vi "Formic Queen.vi"(8 "error in (no error)":errorcluster, 9 "SelfID":i32, 10 "Map":i32[](array[numeric]), 11 "Mother in":refnum<class "Formics.lvclass">) -> (0 "error out":errorcluster, 1 "Direction":T1, 2 "Action":T2, 3 "Mother out":refnum<class "Formics.lvclass">, 4 "Replicated Class":refnum<class "Formics.lvclass">)   [LabVIEW 2015, in "Formics.lvclass"]
uses:
  Formics.lvclass
  Type Defs/Action Enum.ctl
  Type Defs/Direction Enum.ctl
  Formics.lvclass/Formics.ctl
  SquareStatus.ctl
  Formic Types.ctl
  Type Defs/SB Type Defs.lvlib
  Common/Common.lvlib
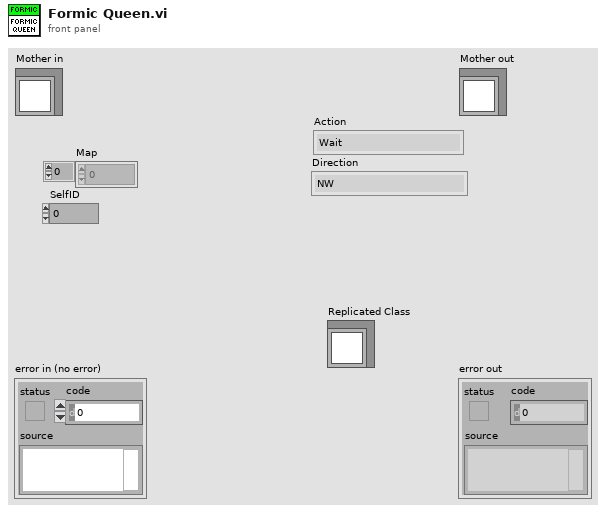
[diagram p1: front panel]
types:
  T1 = typedef "SB Type Defs.lvlib/Direction Enum.ctl" = enum16{"NW", "N", "NE", "E", "SE", "S", "SW", "W"}
  T2 = typedef "SB Type Defs.lvlib/Action Enum.ctl" = enum16{"Wait", "Move", "Attack", "Replicate"}
  T3 = typedef "Formics.lvclass/Formic Types.ctl" = enum16{"Queen Bee", "Protector Bee", "Daughter Bee", "Worker Bee", "Coward"}
  T4 = typedef "Formics.lvclass/SquareStatus.ctl" = cluster{"ID":i32, "Heartbeat":bool, "MyPosition":cluster{"X":i32, "Y":i32}}
  T5 = typedef "Formics.lvclass/Kamikaze DVR.ctl" = refnum<data-value>
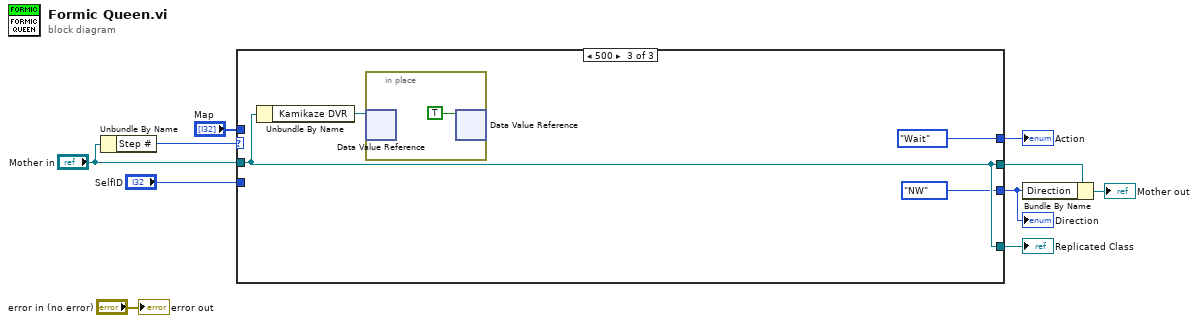
[diagram p0: block diagram]
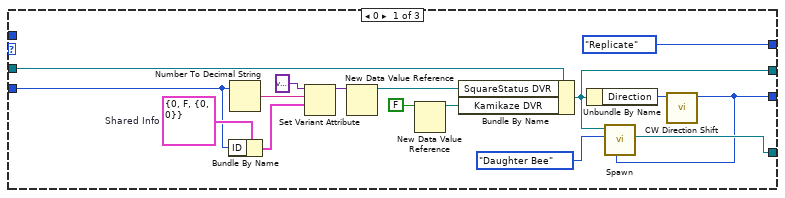
[diagram p2: hidden frame]
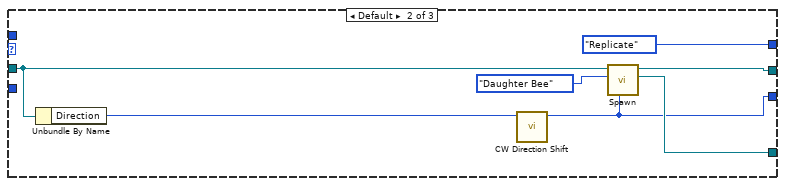
[diagram p3: hidden frame]
diagram:
  n1 = Unbundle By Name("Mother in") -> ("Step #"=w7:i32)
  n2 = case shown="500" w7 {
    tunnel: [w13 w29 w35] -> w9
    tunnel: "Mother in" -> [w18 w30 w35]
    tunnel: "SelfID" -> [w17 _ _]
    tunnel: "Map" -> [_ _ _]
    tunnel: [Action_Enum."Replicate" ("Action") Action_Enum."Replicate" ("Action") Action_Enum."Wait" ("Action")] -> w4
    tunnel: [w12 w28 Direction_Enum."NW" ("Direction")] -> w1
    tunnel: [w15 w31 w35] -> w3
    frame 0 {
      w23 = T4 {"ID"=0, "Heartbeat"=FALSE, "MyPosition"={"X"=0, "Y"=0}}  # Shared Info
      n3 = Bundle By Name(cluster=w23, "ID"=w17) -> (w24:T4)
      n4 = Number To Decimal String(number=w17) -> (decimal integer string=w25:string)  [unwired: 1 in]
      n5 = Set Variant Attribute(Variant=variant ("variant"), name=w25, value=w24) -> (Variant out=w22:variant)  [unwired: 1 in, 2 out]
      n6 = New Data Value Reference(data value=w22) -> (data value reference=w21:refnum<data-value>)  [unwired: 1 in, 1 out]
      n7 = New Data Value Reference(data value=FALSE) -> (data value reference=w20:refnum<data-value>)  [unwired: 1 in, 1 out]
      n8 = Bundle By Name(cluster=w18, "SquareStatus DVR"=w21, "Kamikaze DVR"=w20) -> (w13:refnum<class "Formics.lvclass">)
      n9 = Unbundle By Name(w13) -> ("Direction"=w11:i32)
      n10 = call "CW Direction Shift.vi"("Direction"=w11) -> ("Numeric"=w12:i32)  [unwired: 10 in]
      n11 = call "Spawn.vi"("Start Direction"=w12, "Directive"=Formic_Types."Daughter Bee", "Mother in"=w13) -> ("Replicated Class"=w15:refnum<class "Formics.lvclass">)  [unwired: 6 in, 2 out]
    }
    frame Default {
      n12 = Unbundle By Name(w30) -> ("Direction"=w27:i32)
      n13 = call "CW Direction Shift.vi"("Direction"=w27) -> ("Numeric"=w28:i32)  [unwired: 10 in]
      n14 = call "Spawn.vi"("Start Direction"=w28, "Directive"=Formic_Types."Daughter Bee", "Mother in"=w30) -> ("Replicated Class"=w31:refnum<class "Formics.lvclass">, "Mother out"=w29:refnum<class "Formics.lvclass">)  [unwired: 6 in, 1 out]
    }
    frame 500 {
      n15 = Unbundle By Name(w35) -> ("Kamikaze DVR"=w37:T5)
      n16 = in-place {
        n17 = in-place-dvr #1(w37) -> ()  [unwired: 2 out]
        n18 = in-place-dvr #1(TRUE ("data value")) -> ()  [unwired: 2 out]
      }
    }
  }
  "Action" <- w4
  "Direction" <- w1
  "Replicated Class" <- w3
  n19 = Bundle By Name(cluster=w9, "Direction"=w1) -> (→"Mother out":refnum<class "Formics.lvclass">)
  "error out" <- "error in (no error)"
